vi "M3202 awg gaussian.vi"() -> ()   [LabVIEW 2020]
panel:
  out "errorOut":errorcluster
  in  "amplitude":dbl=1.0
  in  "nChannel":i32=1
  in  "nSlot":i32=3
  in  "nChassis":i32=1
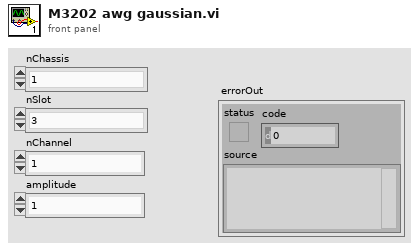
[diagram p1: front panel]
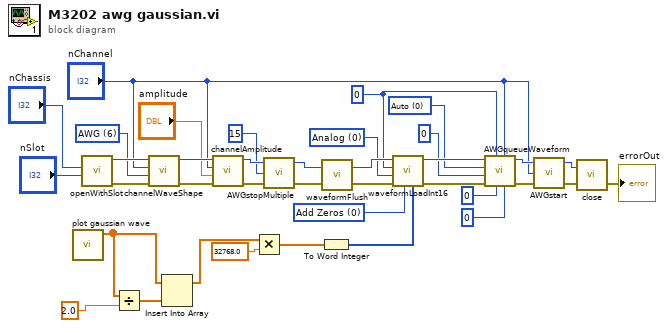
[diagram p0: block diagram]
diagram:
  w15 = 0 items=["Auto"=0, "SW/HVI"=1, "External"=2, "SW/HVI Cycle"=5, "External Cycle"=6] ("triggerMode")
  w12 = 0 ("waveformNumber")
  w17 = 0 items=["Analog"=0, "IQ"=2, "IQ (polar)"=3] ("waveformType")
  w19 = 0 items=["Add Zeros", "Repeat Waveform"] ("paddingMode")
  w33 = 6 items=["HiZ"=-1, "Off"=0, "Sinusoidal"=1, "Triangular"=2, "Sawtooth"=3, "Square"=4, "DC"=5, "AWG"=6, "Partner"=8] ("waveShape")
  n1 = call "plot gaussian wave.vi"() -> ("Array"=w3:dbl[])  [unwired: 11 in]
  n2 = call <vilib>:"openWithSlot.vi"("nSlot"="nSlot", "nChassis"="nChassis") -> ("errorOut"=w35:errorcluster, "moduleID"=w34:i32)  [unwired: 4 in]
  n3 = Divide(x=w3, y=2.0) -> (x/y=w1:dbl[])
  n4 = call <vilib>:"channelWaveShape.vi"("errorIn"=w35, "waveShape"=w33, "nChannel"="nChannel", "moduleID"=w34) -> ("errorOut"=w30:errorcluster, "moduleIDOut"=w32:i32)  [unwired: 2 in]
  n5 = Insert Into Array(array=w3, new element=w1) -> (w4:dbl[])  [unwired: 1 in]
  n6 = call <vilib>:"channelAmplitude.vi"("errorIn"=w30, "amplitude"="amplitude", "nChannel"="nChannel", "moduleID"=w32) -> ("errorOut"=w28:errorcluster, "moduleIDOut"=w29:i32)  [unwired: 2 in]
  n7 = Multiply(x=w4, y=32768.0) -> (x*y=w21:dbl[])
  n8 = call <vilib>:"AWGstopMultiple.vi"("errorIn"=w28, "AWGmask"=15, "moduleID"=w29) -> ("errorOut"=w26:errorcluster, "moduleIDOut"=w27:i32)  [unwired: 1 in]
  n9 = To Word Integer(number=w21) -> (16bit integer=w20:i16[])
  n10 = call <vilib>:"waveformFlush.vi"("errorIn"=w26, "moduleID"=w27) -> ("errorOut"=w18:errorcluster, "moduleIDOut"=w23:i32)
  n11 = call <vilib>:"waveformLoadInt16.vi"("waveformData"=w20, "paddingMode"=w19, "errorIn"=w18, "waveformType"=w17, "waveformNumber"=w12, "moduleID"=w23) -> ("errorOut"=w13:errorcluster, "moduleIDOut"=w16:i32)  [unwired: 3 in, 1 out]
  n12 = call <vilib>:"AWGqueueWaveform.vi"("prescaler"=0, "nAWG"="nChannel", "cycles"=0, "waveformNumber"=w12, "errorIn"=w13, "startDelay"=0, "triggerMode"=w15, "moduleID"=w16) -> ("errorOut"=w7:errorcluster, "moduleIDOut"=w9:i32)  [unwired: 2 in]
  n13 = call <vilib>:"AWGstart.vi"("errorIn"=w7, "nAWG"="nChannel", "moduleID"=w9) -> ("errorOut"=w5:errorcluster, "moduleIDOut"=w6:i32)  [unwired: 1 in]
  n14 = call <vilib>:"close.vi"("errorIn"=w5, "moduleID"=w6) -> ("errorOut"=→"errorOut":errorcluster)  [unwired: 1 in]
